vi "3D-SaveIniConfig.vi"(9 "VISA1":string[](array[string]), 10 "Inputs_BaseParam":string[](array[string]), 11 "名称或相对路径":string="UserDefine.ini") -> ()   [LabVIEW 2017]
uses:
  Global System.vi
  <vilib>/Utility/config.llb/NI_LVConfig.lvlib
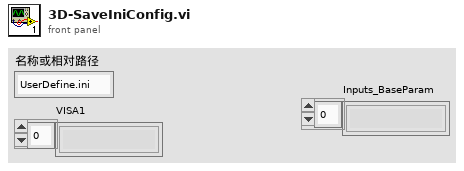
[diagram p1: front panel]
types:
  T1 = typedef "NI_LVConfig.lvlib/Config Data RefNum.ctl" = refnum<k1>
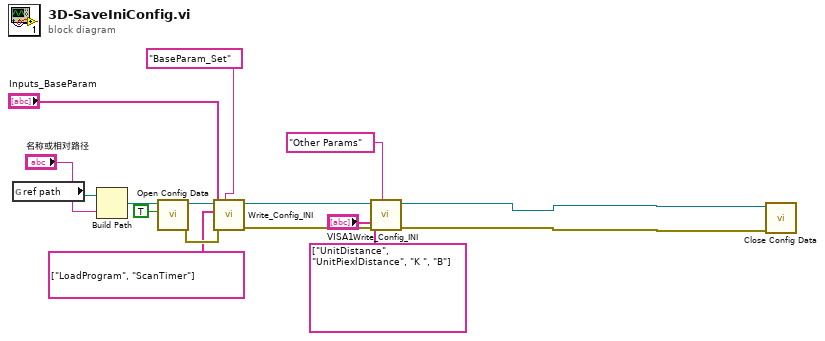
[diagram p0: block diagram]
diagram:
  n1 = global read "Global System.vi" "ref path"() -> (w11:path)
  n2 = Build Path(base path=w11, name or relative path="名称或相对路径") -> (appended path=w9:path)
  n3 = call <vilib>:"Open Config Data.vi"("create file if necessary (T)"=TRUE, "configuration file path"=w9) -> ("error out"=w15:errorcluster, "refnum"=w14:T1)  [unwired: 7 in, 1 out]
  n4 = call "Write_Config_INI.vi"("section"="BaseParam_Set", "error in (no error)"=w15, "Inputs"="Inputs_BaseParam", "Keys"=string[] ["LoadProgram", "ScanTimer"], "refnum"=w14) -> ("error out"=w6:errorcluster, "refnum 2"=w7:T1)  [unwired: 5 in]
  n5 = call "Write_Config_INI.vi"("section"="Other Params", "error in (no error)"=w6, "Inputs"="VISA1", "Keys"=string[] ["UnitDistance", "UnitPiexlDistance", "K ", "B"], "refnum"=w7) -> ("error out"=w4:errorcluster, "refnum 2"=w5:T1)  [unwired: 5 in]
  n6 = call <vilib>:"Close Config Data.vi"("error in (no error)"=w4, "refnum"=w5) -> ()  [unwired: 8 in, 2 out]
